vi "Scan line to grid area.vi"(4 "Y index":u32[](array[numeric]), 5 "X index":u32[](array[numeric]), 6 "Y length":u32, 7 "X length":u32, 8 "Y scan line":u32, 9 "Enable":bool, 10 "Single line scan":i16[](array[numeric]), 11 "Input array":i16[](array[numeric])) -> (3 "Ouput array":i16[](array[numeric]))   [LabVIEW 2018]
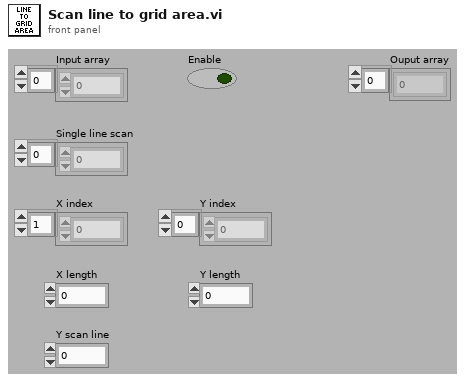
[diagram p1: front panel]
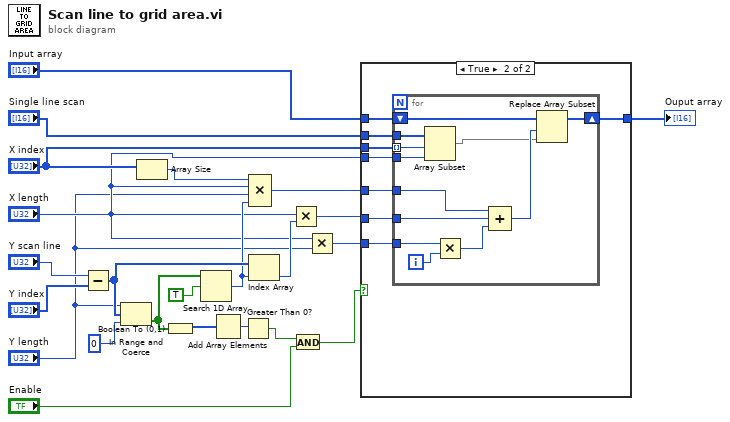
[diagram p0: block diagram]
diagram:
  n1 = Subtract(x="Y scan line", y="Y index") -> (x-y=w15:u32[])
  n2 = In Range and Coerce(upper limit="Y length", x=w15, lower limit=u32 0) -> (In Range?=w19:bool[])  [unwired: 1 out]
  n3 = Array Size(array="X index") -> (size(s)=w13:i32)
  n4 = Boolean To (0,1)(Boolean=w19) -> (0, 1=w20:i16[])
  n5 = Search 1D Array(1D array=w19, element=TRUE) -> (index of element=w14:i32)  [unwired: 1 in]
  n6 = Add Array Elements(numeric array=w20) -> (sum=w22:i16)
  n7 = Greater Than 0?(x=w22) -> (x > 0?=w9:bool)
  n8 = Compound Arithmetic op=MULTIPLY(w13, "X length", "Y length", w14) -> (w12:u32)
  n9 = Index Array(array=w15, index=w14) -> (element=w4:u32)
  n10 = Multiply(x="X length", y=w4) -> (x*y=w3:u32)
  n11 = And(x=w9, y="Enable") -> (x .and. y?=w8:bool)
  n12 = Multiply(x="X length", y="Y length") -> (x*y=w11:u32)
  n13 = case shown="True" w8 {
    tunnel: "Single line scan" -> [_ w32]
    tunnel: "X index" -> [_ w31]
    tunnel: "X length" -> [_ w30]
    tunnel: "Input array" -> [w24 w29]
    tunnel: [w24 w28] -> w10
    tunnel: w12 -> [_ w27]
    tunnel: w11 -> [_ w26]
    tunnel: w3 -> [_ w25]
    frame False {
    }
    frame True {
      n14 = for {
        tunnel: w32 -> [w44]
        tunnel: w31 -> [w43] mode=indexing
        tunnel: w30 -> [w42]
        tunnel: w27 -> [w38]
        tunnel: w26 -> [w34]
        shift-right: [w40] -> w28
        shift-left: w29 -> [w41]
        tunnel: w25 -> [w33]
        i -> [w39]
        n15 = Array Subset(array=w44, index=w43, length=w42) -> (w35:i16[])
        n16 = Multiply(x=w34, y=w39) -> (x*y=w37:u32)
        n17 = Compound Arithmetic op=ADD(w38, w33, w37) -> (w36:u32)
        n18 = Replace Array Subset(array=w41, new element=w35, index=w36) -> (w40:i16[])
      }
    }
  }
  "Ouput array" <- w10
